vi "Get Cold Block Temperature.vi"(8 "error in (no error)":errorcluster, 10 "Storage Index":i32, 11 "Storage Line in":refnum<class "Storage Line.lvclass">) -> (0 "error out":errorcluster, 1 "Temperature (C)":dbl, 2 "Storage Index":i32, 3 "Storage Line out":refnum<class "Storage Line.lvclass">, 4 "Frozen?":bool)   [LabVIEW 2015, in "cRIO-Carbondioxide.lvlib" / "CO2-Actor.lvlib" / "Storage Line.lvclass"]
uses:
  Storage Line.lvclass
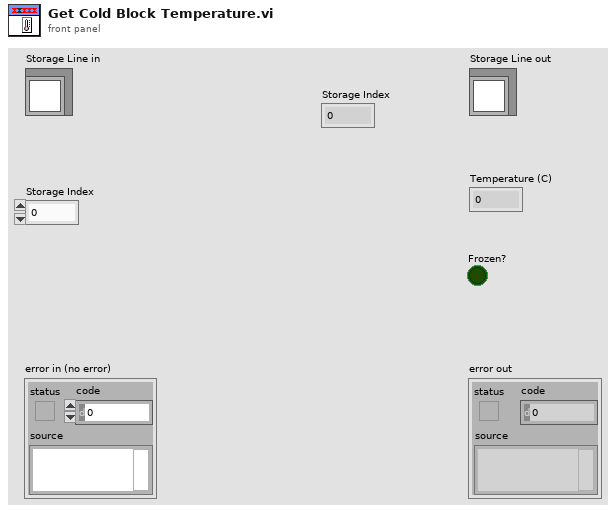
[diagram p1: front panel]
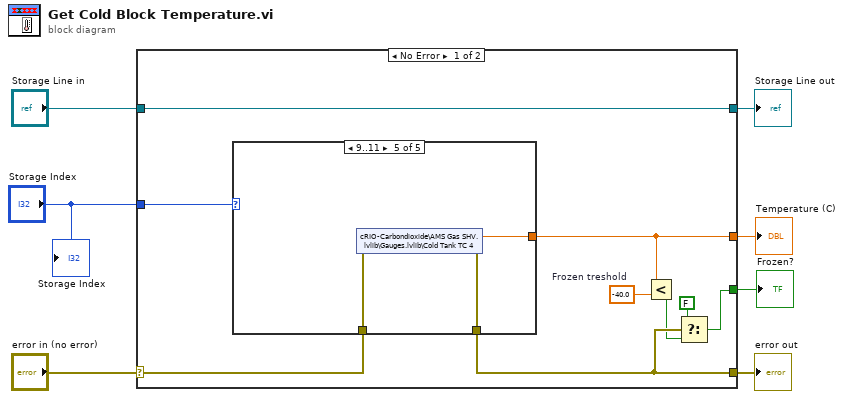
[diagram p0: block diagram]
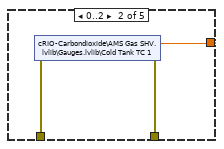
[diagram p3: hidden frame]
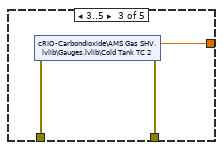
[diagram p4: hidden frame]
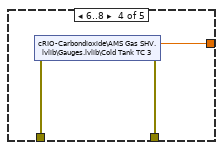
[diagram p5: hidden frame]
diagram:
  n1 = case shown="No Error" "error in (no error)" {
    selector: "error in (no error)" -> [w14 w31]
    tunnel: [w11 w31] -> w6
    tunnel: [w16 w30] -> w4
    tunnel: "Storage Line in" -> [w16 w30]
    tunnel: "Storage Index" -> [w15 _]
    tunnel: [w13 _] -> w2
    tunnel: [w9 _] -> w1
    frame No Error {
      w12 = -40.0  # Frozen treshold
      n2 = case shown="9..11" w15 {
        tunnel: w14 -> [w17 w20 w23 w26 w29]
        tunnel: [w17 w19 w22 w25 w28] -> w11
        tunnel: [_ w18 w21 w24 w27] -> w13
        frame -1, Default {
        }
        frame 0..2 {
          n3 = shared-variable "cRIO-Carbondioxide\\AMS Gas SHV.lvlib\\Gauges.lvlib\\Cold Tank TC 1"(error in=w20) -> (w18:dbl, error out=w19:errorcluster)
        }
        frame 3..5 {
          n4 = shared-variable "cRIO-Carbondioxide\\AMS Gas SHV.lvlib\\Gauges.lvlib\\Cold Tank TC 2"(error in=w23) -> (w21:dbl, error out=w22:errorcluster)
        }
        frame 6..8 {
          n5 = shared-variable "cRIO-Carbondioxide\\AMS Gas SHV.lvlib\\Gauges.lvlib\\Cold Tank TC 3"(error in=w26) -> (w24:dbl, error out=w25:errorcluster)
        }
        frame 9..11 {
          n6 = shared-variable "cRIO-Carbondioxide\\AMS Gas SHV.lvlib\\Gauges.lvlib\\Cold Tank TC 4"(error in=w29) -> (w27:dbl, error out=w28:errorcluster)
        }
      }
      n7 = Less?(x=w13, y=w12) -> (x < y?=w10:bool)
      n8 = Select(t=FALSE, s=w11, f=w10) -> (s? t:f=w9:bool)
    }
    frame Error {
    }
  }
  "error out" <- w6
  "Storage Line out" <- w4
  "Temperature (C)" <- w2
  "Frozen?" <- w1
  "Storage Index" <- "Storage Index"
